vi "editscenario handle import.vi"(6 "User Information":T2, 7 "Connection Refnum":T1, 8 "error in (no error)":errorcluster, 11 "Scenario XML (\"\")":string) -> (0 "error out":errorcluster, 3 "Scenario Record":T3, 5 "dup Connection Ref":T1)   [LabVIEW 2011]
uses:
  server/database/Scenarios/Scenario Record.ctl
  server/database/Scenarios/Conditions/Condition Record.ctl
  server/database/Scenarios/Conditions/Condition Operators.ctl
  server/database/Users/User Record.ctl
  Summitek EXT/ODBC/SQL Controls/Connection Refnum.ctl
  scenario xml.ctl
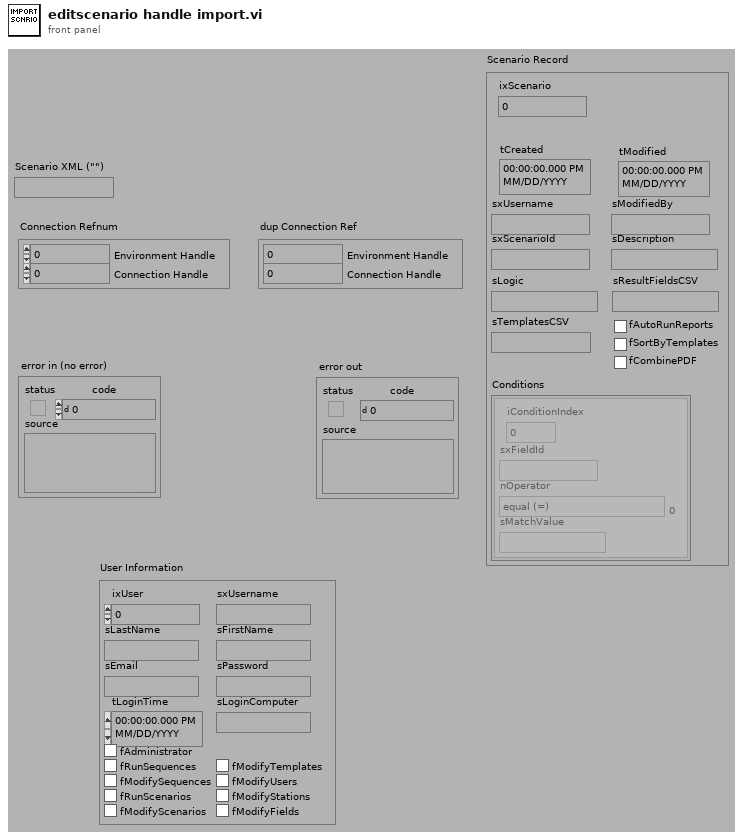
[diagram p1: front panel]
types:
  T1 = typedef "Connection Refnum.ctl" = cluster{"Environment Handle":i32, "Connection Handle":i32}
  T2 = typedef "User Record.ctl" = cluster{"ixUser":i32, "sxUsername":string, "sLastName":string, "sFirstName":string, "sEmail":string, "sPassword":string, "tLoginTime":timestamp, "sLoginComputer":string, "fAdministrator":bool, "fRunSequences":bool, "fModifySequences":bool, "fRunScenarios":bool, "fModifyScenarios":bool, "fModifyTemplates":bool, "fModifyUsers":bool, "fModifyStations":bool, "fModifyFields":bool}
  T3 = typedef "Scenario Record.ctl" = cluster{"ixScenario":i32, "tCreated":timestamp, "tModified":timestamp, "sxUsername":string, "sModifiedBy":string, "sxScenarioId":string, "sDescription":string, "sLogic":string, "sResultFieldsCSV":string, "sTemplatesCSV":string, "fAutoRunReports":bool, "fSortByTemplates":bool, "fCombinePDF":bool, "Conditions":T4[]}
  T4 = typedef "Condition Record.ctl" = cluster{"iConditionIndex":i32, "sxFieldId":string, "nOperator":T5, "sMatchValue":string}
  T5 = typedef "Condition Operators.ctl" = enum16{"equal (=)", "not equal (\\u2260)", "less than (<)", "less than or equal (\\u2264)", "greater than (>)", "greater than or equal (\\u2265)", "contains", "does not contain"}
  T6 = typedef "scenario xml.ctl" = cluster{"#attributes":cluster{"version":string, "creator":string}, "sxScenarioId":string, "sDescription":string, "sLogic":string, "sResultFieldsCSV":string, "sTemplatesCSV":string, "fAutoRunReports":bool, "fSortByTemplates":bool, "fCombinePDF":bool, "Conditions":cluster{"sxFieldId":string, "nOperator":string, "sMatchValue":string}[]}
  T7 = cluster{"sxFieldId":string, "nOperator":string, "sMatchValue":string}[]
  T8 = typedef "Field Record.ctl" = cluster{"ixField":i32, "iSequenceOrder":i32, "sxFieldId":string, "sxSequenceId":string, "sDisplayName":string, "sValue":string, "sUnits":string, "nDataType":T9, "nNextItem":T10, "fSystem":bool, "fSystemValue":bool, "fRequired":bool, "fSetAtTest":bool, "fTestField":bool, "fDeleted":bool, "fIndexed":bool, "fFreeList":bool}
  T9 = typedef "Field DataTypes.ctl" = enum32{"text", "numeric", "list", "timestamp", "boolean"}
  T10 = typedef "Field NextItem.ctl" = enum32{"Reset", "Retain", "Auto-Increment"}
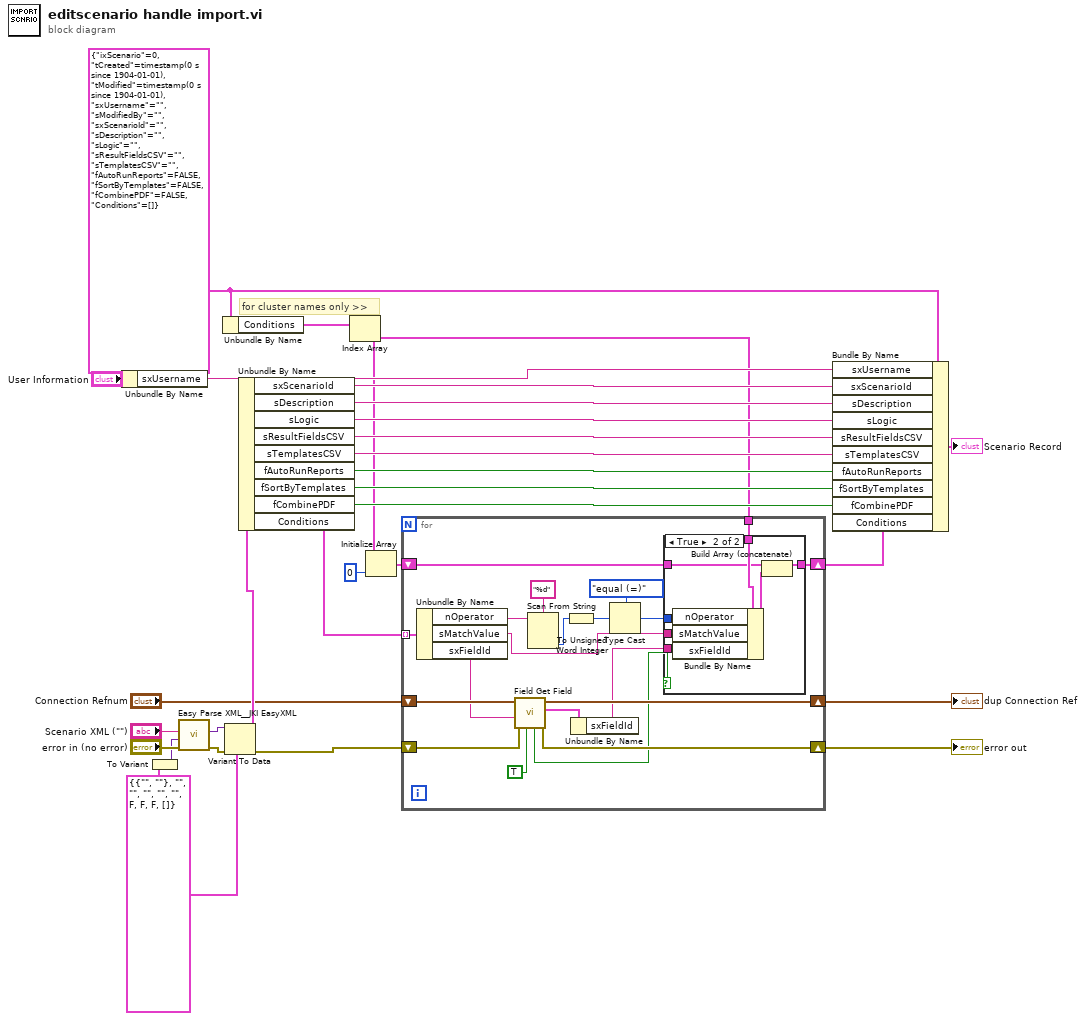
[diagram p0: block diagram]
diagram:
  w16 = T3 {"ixScenario"=0, "tCreated"=timestamp(0 s since 1904-01-01), "tModified"=timestamp(0 s since 1904-01-01), "sxUsername"="", "sModifiedBy"="", "sxScenarioId"="", "sDescription"="", "sLogic"="", "sResultFieldsCSV"="", "sTemplatesCSV"="", "fAutoRunReports"=FALSE, "fSortByTemplates"=FALSE, "fCombinePDF"=FALSE, "Conditions"=[]} ("Scenario Record")
  w2 = T6 {"#attributes"={"version"="", "creator"=""}, "sxScenarioId"="", "sDescription"="", "sLogic"="", "sResultFieldsCSV"="", "sTemplatesCSV"="", "fAutoRunReports"=FALSE, "fSortByTemplates"=FALSE, "fCombinePDF"=FALSE, "Conditions"=[]} ("scenario")
  # "for cluster names only >>"
  n1 = Unbundle By Name("User Information") -> ("sxUsername"=w14:string)
  n2 = To Variant(anything=w2) -> (Variant=w21:variant)
  n3 = call "Easy Parse XML__JKI EasyXML.vi"("error in (no error)"="error in (no error)", "LabVIEW Data (Type)"=w21, "XML String"="Scenario XML (\"\")") -> ("error out"=w20:errorcluster, "LabVIEW Data"=w19:variant)  [unwired: 7 out]
  n4 = Unbundle By Name(w16) -> ("Conditions"=w24:T4[])
  n5 = Variant To Data(error in=w20, type=w2, Variant=w19) -> (data=w18:T6, error out=w12:errorcluster)
  n6 = Unbundle By Name(w18) -> ("sxScenarioId"=w29:string, "sDescription"=w28:string, "sLogic"=w27:string, "sResultFieldsCSV"=w26:string, "sTemplatesCSV"=w23:string, "fAutoRunReports"=w3:bool, "fSortByTemplates"=w5:bool, "fCombinePDF"=w4:bool, "Conditions"=w25:T7)
  n7 = Index Array(array=w24) -> (element=w1:T4)  [unwired: 1 in]
  n8 = Initialize Array(w1, 0 ("dimension size")) -> (w7:T4[])
  n9 = for {
    tunnel: w25 -> [w49] mode=indexing
    tunnel: w1 -> [w48]
    shift-right: [w39] -> w11
    shift-left: w12 -> [w40]
    shift-right: [w37] -> w9
    shift-left: "Connection Refnum" -> [w38]
    shift-right: [w30] -> w6
    shift-left: w7 -> [w31]
    n10 = Unbundle By Name(w49) -> ("nOperator"=w45:string, "sMatchValue"=w47:string, "sxFieldId"=w35:string)
    n11 = call "Field Get Field.vi"("by sDisplayName? (f, by sFieldId)"=TRUE, "error in (no error)"=w40, "sFieldId or sDisplayName (\"\")"=w35, "Connection Refnum"=w38) -> ("error out"=w39:errorcluster, "Field"=w33:T8, "Connection Refnum"=w37:T1, "Data Present?"=w34:bool)  [unwired: 1 in, 3 out]
    n12 = Scan From String(format string="%d", input string=w45) -> (output 1=w44:i32)  [unwired: 2 in, 4 out]
    n13 = To Unsigned Word Integer(number=w44) -> (unsigned 16bit integer=w42:u16)
    n14 = Unbundle By Name(w33) -> ("sxFieldId"=w32:string)
    n15 = Type Cast(type=Condition_Operators."equal (=)" ("nOperator"), x=w42) -> (*(type *) &x=w41:T5)
    n16 = case shown="True" w34 {
      tunnel: w48 -> [_ w57]
      tunnel: w47 -> [_ w56]
      tunnel: w41 -> [_ w55]
      tunnel: w32 -> [_ w54]
      tunnel: w31 -> [w50 w52]
      tunnel: [w50 w51] -> w30
      frame False {
      }
      frame True {
        n17 = Bundle By Name(cluster=w57, "nOperator"=w55, "sMatchValue"=w56, "sxFieldId"=w54) -> (w53:T4)
        n18 = Build Array (concatenate)(w52, w53) -> (w51:T4[])
      }
    }
  }
  "error out" <- w11
  "dup Connection Ref" <- w9
  n19 = Bundle By Name(cluster=w16, "sxUsername"=w14, "sxScenarioId"=w29, "sDescription"=w28, "sLogic"=w27, "sResultFieldsCSV"=w26, "sTemplatesCSV"=w23, "fAutoRunReports"=w3, "fSortByTemplates"=w5, "fCombinePDF"=w4, "Conditions"=w6) -> (→"Scenario Record":T3)
